vi "Execute.vi"(8 "error in (no error)":errorcluster, 10 "Abstract Producer in":refnum<class "Abstract Producer.lvclass">, 11 "Abstract Response Message in":refnum<class "Abstract Response Message.lvclass">) -> (0 "error out":errorcluster, 2 "Abstract Producer out":refnum<class "Abstract Producer.lvclass">, 3 "Abstract Response Message out":refnum<class "Abstract Response Message.lvclass">)   [LabVIEW 2017, in "Messaging.lvlib" / "Abstract Response Message.lvclass"]
uses:
  Abstract Response Message.lvclass
  Producer/Abstract Producer/Abstract Producer.lvclass
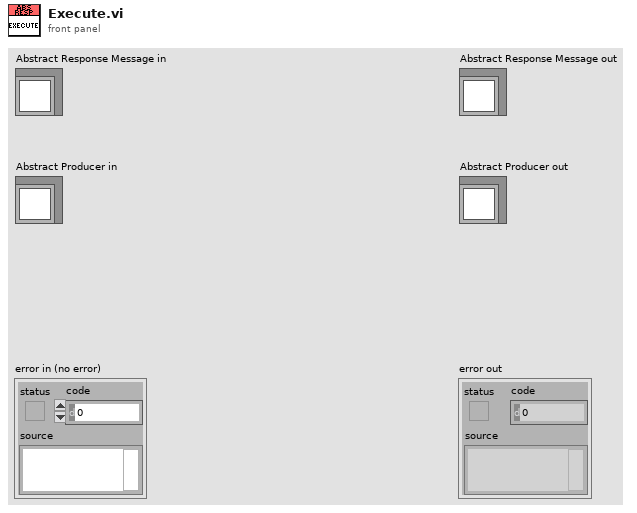
[diagram p1: front panel]
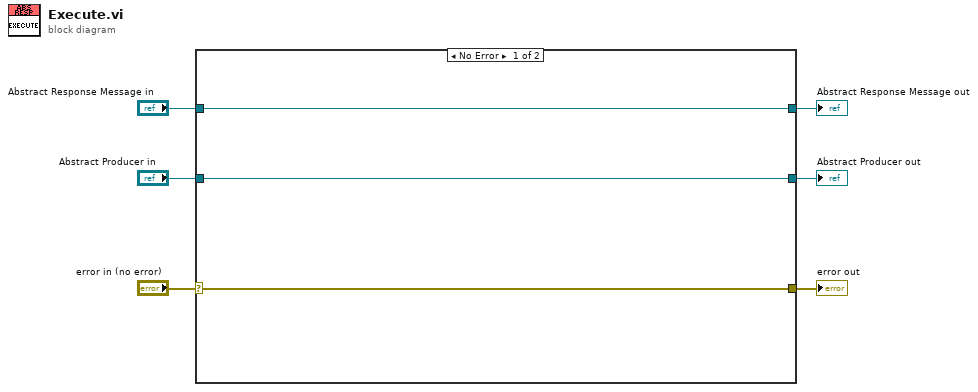
[diagram p0: block diagram]
diagram:
  n1 = case shown="No Error" "error in (no error)" {
    selector: "error in (no error)" -> [w8 w12]
    tunnel: [w8 w12] -> w5
    tunnel: [w9 w11] -> w3
    tunnel: "Abstract Response Message in" -> [w9 w11]
    tunnel: [w7 w10] -> w2
    tunnel: "Abstract Producer in" -> [w7 w10]
    frame No Error {
    }
    frame Error {
    }
  }
  "error out" <- w5
  "Abstract Response Message out" <- w3
  "Abstract Producer out" <- w2
